vi "for_v0_v21.vi"() -> ()   [LabVIEW 2009]
panel:
  in  "X maxim":dbl=4.0
  in  "stop":bool
  out "Graficul functiei e^x":dbl[](graph)=[1.0, 1.137726824439093, 1.2944223270482627, 1.472699003635681, 1.6755291607610396, 1.906294471327756, 2.1688423553095277, 2.4675501256153116, 2.807397968560594, 3.194051975707205, 3.6339586114147693, 4.134452191108021, 4.703877162184579, 5.351727226283833, 6.088803622424141, 6.927395209973865, 7.881483353878148, 8.966975028077357, 10.201968023519097, 11.607052682427556, 13.205655189475557, 15.024428143359653, 17.093694920557923, 19.447955239897016, 22.126460356921648, 25.173867477957945, 28.640984304547647, 32.58561612162291, 37.07352955244534, 42.17954904845251, 47.98880439516885]
  in  "Numar de puncte":u8(slide)=31 scale=0.0..100.0
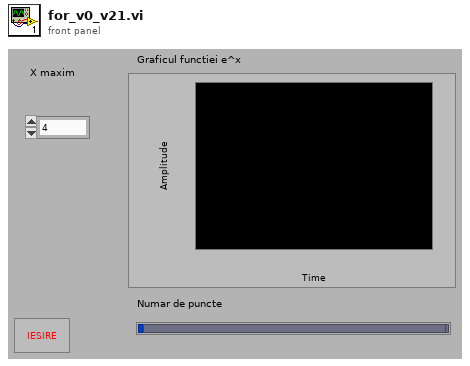
[diagram p1: front panel]
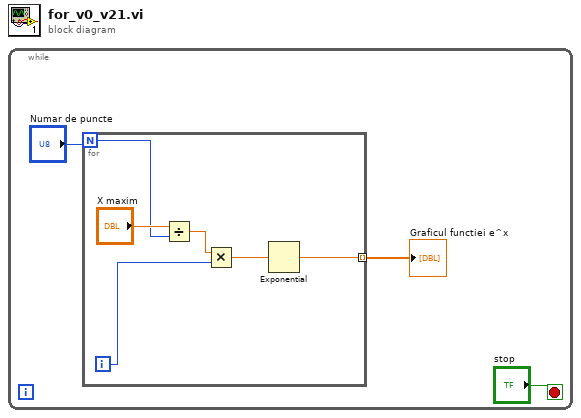
[diagram p0: block diagram]
diagram:
  n1 = while {
    stop <- "stop" stop-if-true
    n2 = for {
      N: "Numar de puncte" -> [w4]
      tunnel: [w9] -> w3 mode=indexing
      i -> [w8]
      n3 = Divide(x="X maxim", y=w4) -> (x/y=w6:dbl)
      n4 = Multiply(x=w6, y=w8) -> (x*y=w7:dbl)
      n5 = Exponential(1:w7) -> (0:w9:dbl)
    }
    "Graficul functiei e^x" <- w3
  }
